vi "CAEN_HVBoard.ProcCases.vi"(0 "i ref in":refnum<vi>, 1 "selector":string, 2 "Data":T1, 3 "call cluster":T2={"Object"="", "Selector"="", "CallType"=enum."synchronous", "Async Object"="", "Async Selector"="", "Data Descriptor"="", "Data"=[], "Error #"=0, "Expire"=0}, 5 "error in (no error)":errorcluster) -> (14 "i ref out":refnum<vi>, 17 "answer cluster":T2={"Object"="", "Selector"="", "CallType"=enum."synchronous", "Async Object"="", "Async Selector"="", "Data Descriptor"="", "Data"=[], "Error #"=0, "Expire"=0}, 19 "error out":errorcluster)   [LabVIEW 2014, in "CAEN_HVBoard.lvlib"]
doc: "This method is called by a process from within the default case in the event loop. The methods of a class that are linked to events will be called from THIS method. Add your code here."
uses:
  CAEN_HVBoard.lvlib
  CSCore/CSSystem/CoreDefs/CoreDefs.call_type.ctl
  CSCore/BaseProcess/BaseProcess.descriptor string definition.ctl
  CSCore/CSSystem/CoreDefs/CoreDefs.rawDataType.ctl
  CSCore/CSApplicationBaseClasses/DeviceBase/DeviceBase.deviceState.ctl
  CSCore/CSSystem/CoreLib/CoreLib.string 2 byte array.vi
  CSCore/CSSystem/CoreLib/CoreLib.byte array 2 string.vi
  CSCore/CSSystem/CoreLib/CoreLib.lvlib
  CSCore/BaseProcess/BaseProcess.lvlib
  CSCore/CSApplicationBaseClasses/DeviceBase/DeviceBase.lvlib
  CSCore/CAEObj/CAEObj.lvlib
  CAEN_HVSystem/CAEN_HVSystem.lvlib
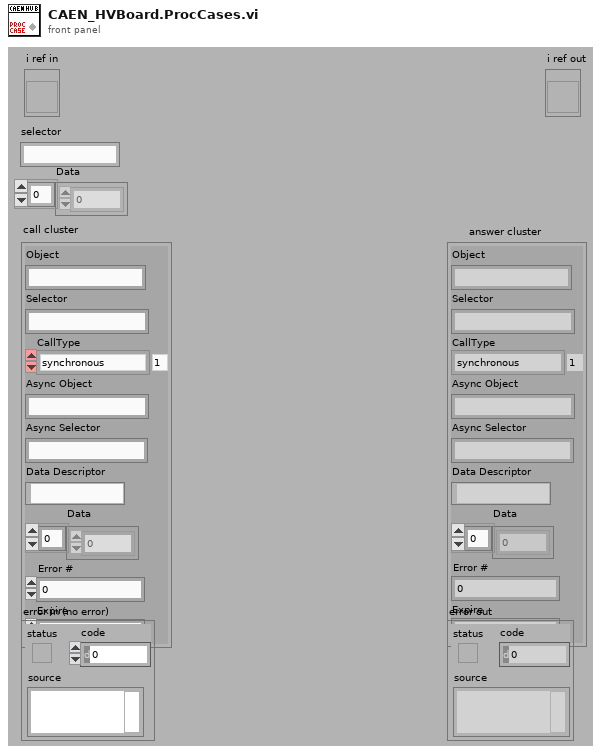
[diagram p1: front panel]
types:
  T1 = typedef "CoreDefs.rawDataType.ctl" = i8[]
  T2 = typedef "CoreDefs.call_type.ctl" = cluster{"Object":string, "Selector":string, "CallType":enum16{"simple", "synchronous", "asynchronous"}, "Async Object":string, "Async Selector":string, "Data Descriptor":T3, "Data":T1, "Error #":i32, "Expire":u32}
  T3 = typedef "BaseProcess.lvlib/BaseProcess.descriptor string definition.ctl" = string
  T4 = typedef "CAEN_HVBoard.lvlib/CAEN_HVBoard.i attribute.ctl" = cluster{"System Name":string, "Board ID":i32, "Prefix":string, "HVMaxMultiplier":dbl, "Temp#Multiplier":dbl, "Model Name":cluster{"Model Name":string, "DIM Status":cluster{"no link":bool, "quality":i32, "Time Stamp":timestamp}}, "Description":cluster{"Description":string, "DIM Status":cluster{"no link":bool, "quality":i32, "Time Stamp":timestamp}}, "SerNum":cluster{"SerNum":i16, "DIM Status":cluster{"no link":bool, "quality":i32, "Time Stamp":timestamp}}, "NrOfCh":cluster{"NrOfCh":i16, "DIM Status":cluster{"no link":bool, "quality":i32, "Time Stamp":timestamp}}, "BdStatus":cluster{"BdStatus":i16, "DIM Status":cluster{"no link":bool, "quality":i32, "Time Stamp":timestamp}}, "HVMax":cluster{"HVMax":dbl, "DIM Status":cluster{"no link":bool, "quality":i32, "Time Stamp":timestamp}}, "HVMax#EU":cluster{"HVMax#EU":string, "DIM Status":cluster{"no link":bool, "quality":i32, "Time Stamp":timestamp}}, "HVMax#HighEU":cluster{"HVMax#HighEU":dbl, "DIM Status":cluster{"no link":bool, "quality":i32, "Time Stamp":timestamp}}, "HVMax#LowEU":cluster{"HVMax#LowEU":dbl, "DIM Status":cluster{"no link":bool, "quality":i32, "Time Stamp":timestamp}}, "Temp#EU":cluster{"Temp#EU":string, "DIM Status":cluster{"no link":bool, "quality":i32, "Time Stamp":timestamp}}, "Temp":cluster{"Temp":dbl, "DIM Status":cluster{"no link":bool, "quality":i32, "Time Stamp":timestamp}}, "Temp#HighEU":cluster{"Temp#HighEU":dbl, "DIM Status":cluster{"no link":bool, "quality":i32, "Time Stamp":timestamp}}, "Temp#LowEU":cluster{"Temp#LowEU":dbl, "DIM Status":cluster{"no link":bool, "quality":i32, "Time Stamp":timestamp}}}
  T5 = typedef "DeviceBase.lvlib/DeviceBase.i attribute.ctl" = cluster{"deviceState":i32, "deviceStateID":i32, "deviceID":string, "deviceIDID":i32, "advancedGUIClass":string, "advancedGUIClassID":i32}
  T6 = typedef "DeviceBase.lvlib/DeviceBase.deviceState.ctl" = i16
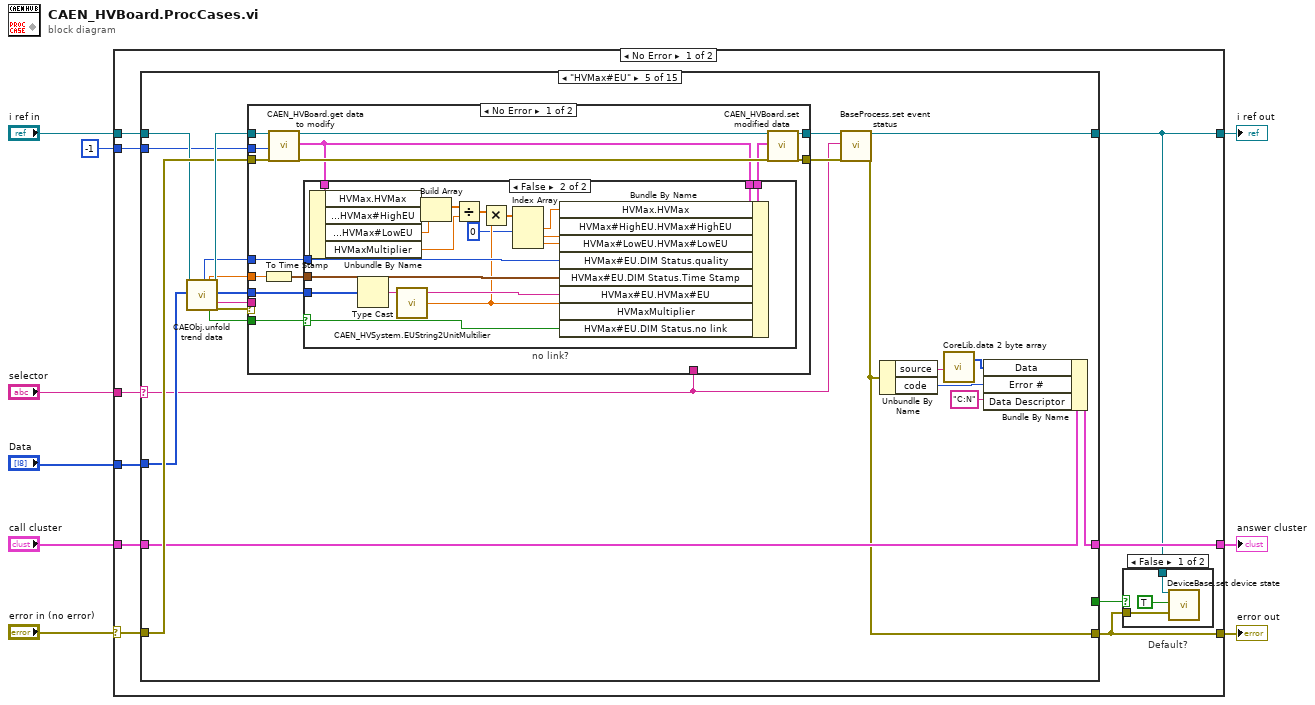
[diagram p0: block diagram]
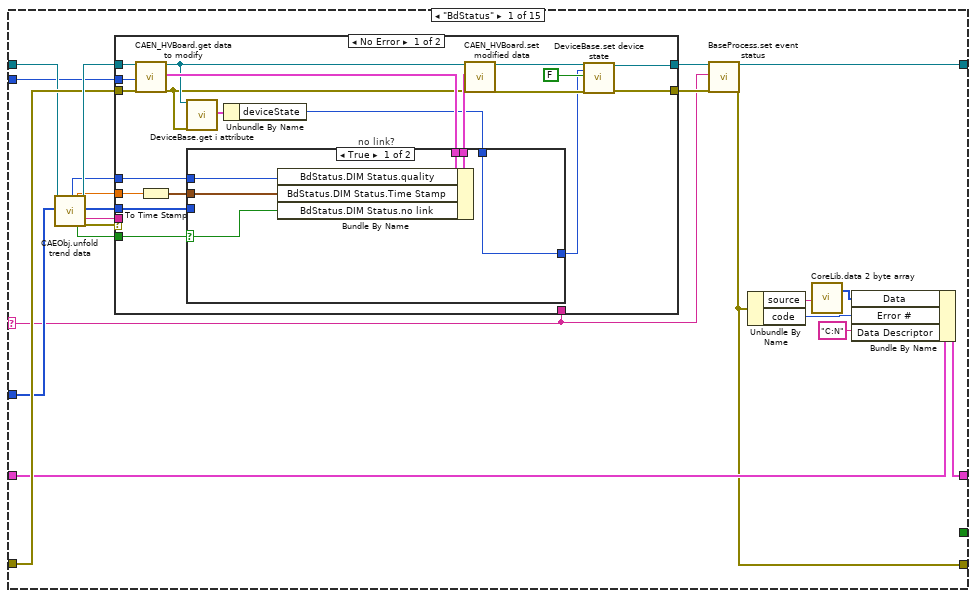
[diagram p3: hidden frame]
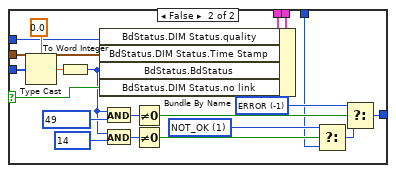
[diagram p4: hidden frame]
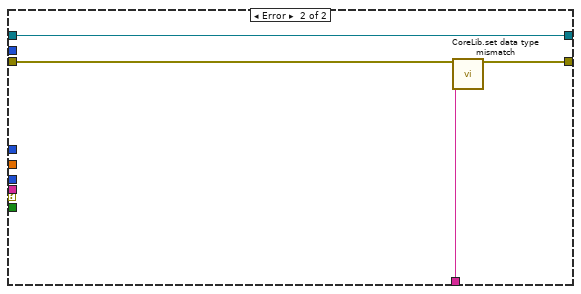
[diagram p5: hidden frame]
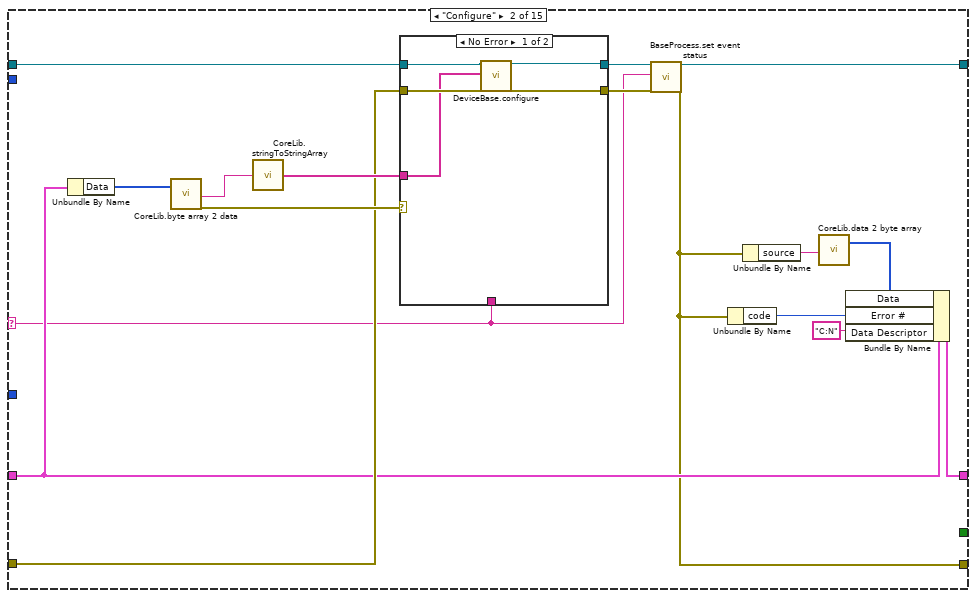
[diagram p6: hidden frame]
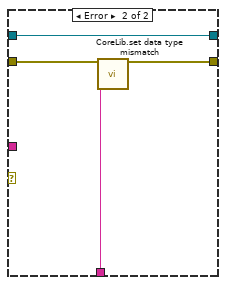
[diagram p7: hidden frame]
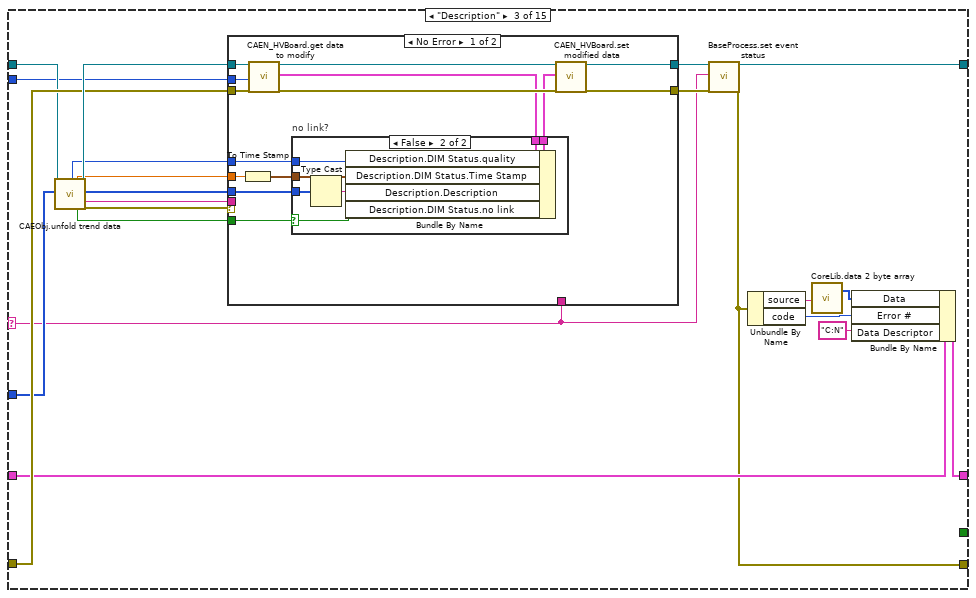
[diagram p8: hidden frame]
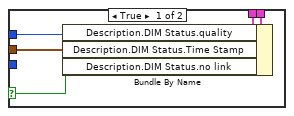
[diagram p9: hidden frame]
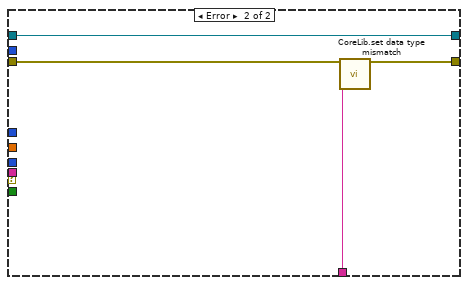
[diagram p10: hidden frame]
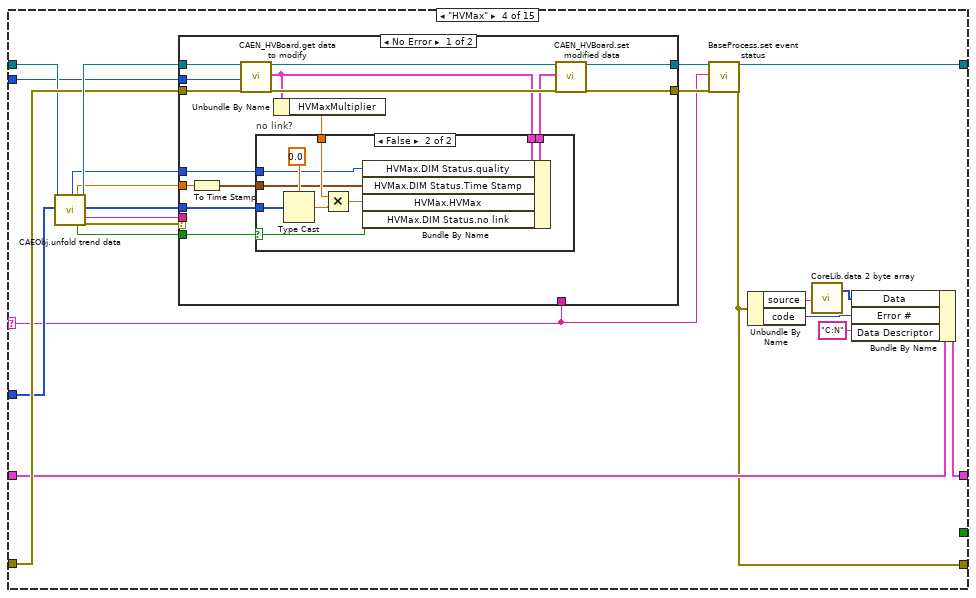
[diagram p11: hidden frame]
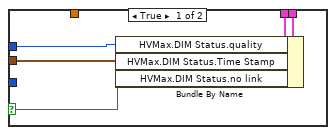
[diagram p12: hidden frame]
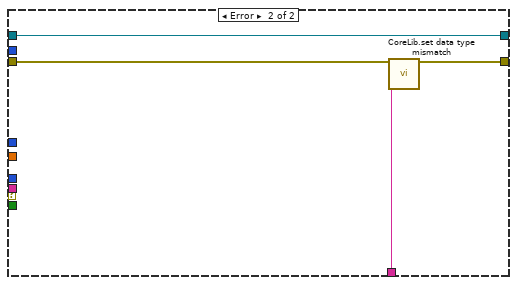
[diagram p13: hidden frame]
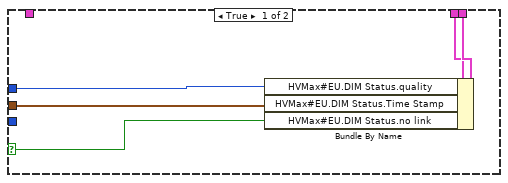
[diagram p14: hidden frame]
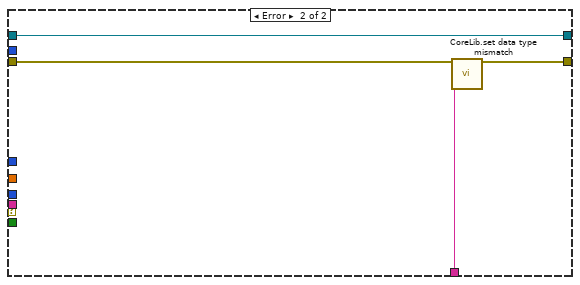
[diagram p15: hidden frame]
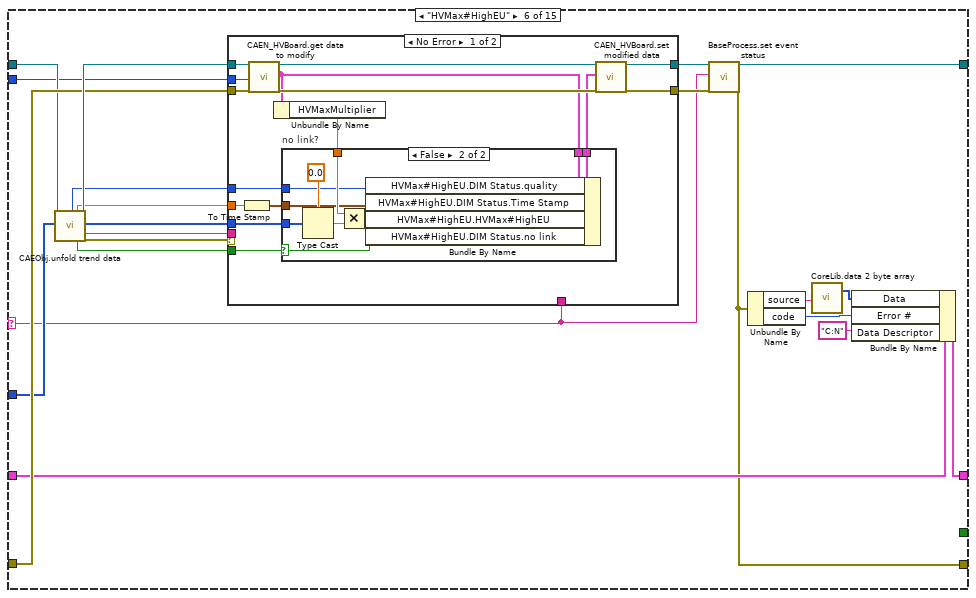
[diagram p16: hidden frame]
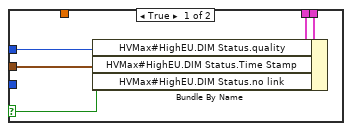
[diagram p17: hidden frame]
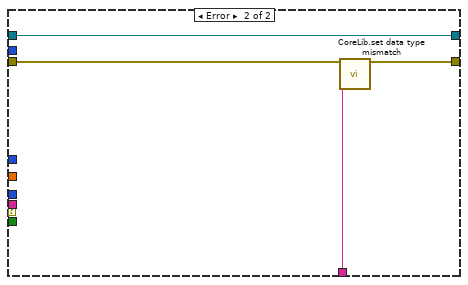
[diagram p18: hidden frame]
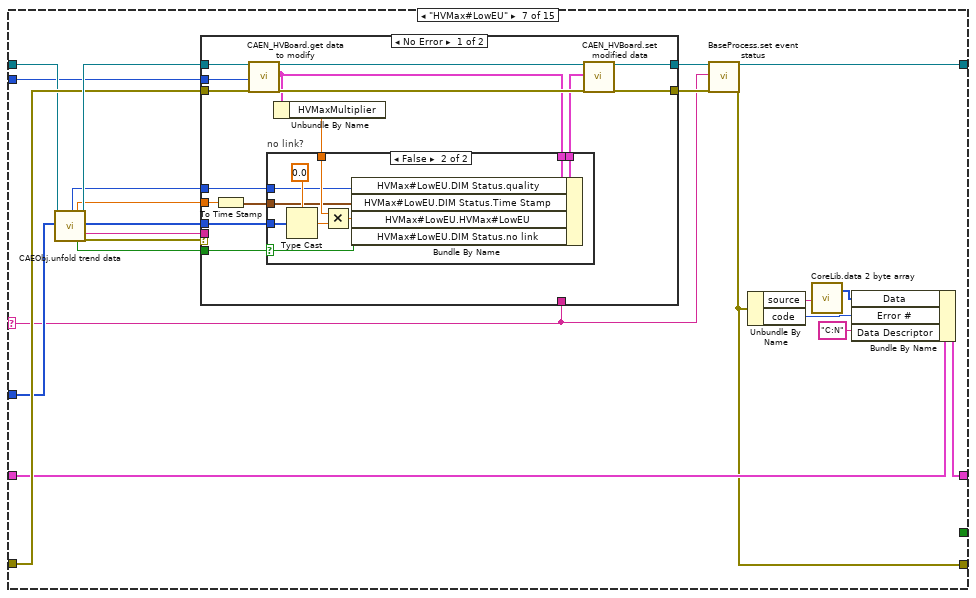
[diagram p19: hidden frame]
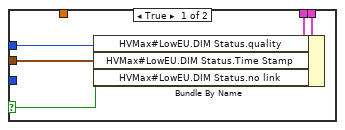
[diagram p20: hidden frame]
diagram:
  n1 = case shown="No Error" "error in (no error)" {
    selector: "error in (no error)" -> [w14 w848]
    tunnel: "selector" -> [w19 _]
    tunnel: [w18 w849] -> w8
    tunnel: "Data" -> [w17 _]
    tunnel: "call cluster" -> [w16 w849]
    tunnel: "i ref in" -> [w15 w850]
    tunnel: [w10 w850] -> w4
    tunnel: [w12 w848] -> w3
    tunnel: -1 ("ms timeout (10000)") -> [w11 _]
    frame No Error {
      n2 = case shown="\"HVMax#EU\"" w19 {
        selector: w19 -> [w32 w99 w129 w181 w237 w303 w359 w415 w487 w541 w615 w671 w737 w793 w842]
        tunnel: w17 -> [w33 _ w130 w182 w238 w304 w360 w416 w488 w542 w616 w672 w738 w794 _]
        tunnel: w15 -> [w31 w98 w128 w180 w236 w302 w358 w414 w486 w540 w614 w670 w736 w792 w841]
        tunnel: [w27 w97 w124 w176 w232 w298 w354 w410 w482 w536 w610 w666 w732 w788 w847] -> w10
        tunnel: w16 -> [w34 w100 w131 w183 w239 w305 w361 w417 w489 w543 w617 w673 w739 w795 w843]
        tunnel: [w28 w96 w125 w177 w233 w299 w355 w411 w483 w537 w611 w667 w733 w789 w844] -> w18
        tunnel: w14 -> [w35 w101 w132 w184 w240 w306 w362 w418 w490 w544 w618 w674 w740 w796 w846]
        tunnel: [w29 w95 w126 w178 w234 w300 w356 w412 w484 w538 w612 w668 w734 w790 w845] -> w12
        tunnel: [_ _ _ _ _ _ _ _ _ _ _ _ _ _ TRUE] -> w13
        tunnel: w11 -> [w30 _ w127 w179 w235 w301 w357 w413 w485 w539 w613 w669 w735 w791 _]
        frame "BdStatus" {
          n3 = call "CAEObj.unfold trend data.vi"("i ref in"=w31, "raw trend data"=w33) -> ("quality"=w26:i32, "timeStamp"=w25:dbl, "no link"=w23:bool, "i ref out"=w39:refnum<vi>, "data"=w38:i8[], "typeDescriptor"=w36:string, "error out"=w24:errorcluster)  [unwired: 9 in, 2 out]
          n4 = case shown="No Error" w24 {
            tunnel: [w48 w94] -> w42
            tunnel: w39 -> [w64 w94]
            tunnel: w35 -> [w63 w93]
            tunnel: [w47 w92] -> w41
            tunnel: w32 -> [_ w91]
            tunnel: w30 -> [w62 _]
            tunnel: w38 -> [w60 _]
            tunnel: w36 -> [_ _]
            tunnel: w26 -> [w58 _]
            tunnel: w25 -> [w56 _]
            tunnel: w23 -> [w55 _]
            frame No Error {
              n5 = call "CAEN_HVBoard.get data to modify.vi"("i ref in"=w64, "ms timeout (10000)"=w62, "error in (no error)"=w63) -> ("i ref out"=w53:refnum<vi>, "i attribute"=w59:T4, "error out"=w52:errorcluster)  [unwired: 13 in, 1 out]
              n6 = To Time Stamp(1:w56) -> (0:w57:timestamp)
              n7 = call "DeviceBase.get i attribute.vi"("i ref in"=w53, "error in (no error)"=w52) -> ("i attribute"=w54:T5)  [unwired: 15 in, 2 out]
              n8 = Unbundle By Name(w54) -> ("deviceState"=w45:i32)
              n9 = case "no link?" shown="True" w55 {
                selector: w55 -> [w66 w83]
                tunnel: [w70 w90] -> w61
                tunnel: w60 -> [_ w89]
                tunnel: w59 -> [w69 w88]
                tunnel: w58 -> [w68 w85]
                tunnel: w57 -> [w67 w84]
                tunnel: [w65 w79] -> w46
                tunnel: w45 -> [w65 w71]
                frame True {
                  n10 = Bundle By Name(cluster=w69, "BdStatus.DIM Status.quality"=w68, "BdStatus.DIM Status.Time Stamp"=w67, "BdStatus.DIM Status.no link"=w66) -> (w70:T4)
                }
                frame False {
                  w73 = T6 1 items=["ERROR"=-1, "OK"=0, "NOT_OK"=1] ("deviceState")
                  w82 = T6 -1 items=["ERROR"=-1, "OK"=0, "NOT_OK"=1] ("deviceState")
                  n11 = Type Cast(type=0.0, x=w89) -> (*(type *) &x=w87:dbl)
                  n12 = To Word Integer(number=w87) -> (16bit integer=w76:i16)
                  n13 = Bundle By Name(cluster=w88, "BdStatus.DIM Status.quality"=w85, "BdStatus.DIM Status.Time Stamp"=w84, "BdStatus.BdStatus"=w76, "BdStatus.DIM Status.no link"=w83) -> (w90:T4)
                  n14 = And(x=w76, y=i16 49) -> (x .and. y?=w81:i16)
                  n15 = And(x=w76, y=i16 14) -> (x .and. y?=w78:i16)
                  n16 = Not Equal To 0?(x=w81) -> (x != 0?=w80:bool)
                  n17 = Not Equal To 0?(x=w78) -> (x != 0?=w74:bool)
                  n18 = Select(t=w73, s=w74, f=w71) -> (s? t:f=w72:i32)
                  n19 = Select(t=w82, s=w80, f=w72) -> (s? t:f=w79:i32)
                }
              }
              n20 = call "CAEN_HVBoard.set modified data.vi"("i ref in"=w53, "i attribute"=w61, "error in (no error)"=w52) -> ("i ref out"=w49:refnum<vi>, "error out"=w50:errorcluster)  [unwired: 15 in]
              n21 = call "DeviceBase.set device state.vi"("i ref in"=w49, "deviceState"=w46, "implicit"=FALSE, "error in (no error)"=w50) -> ("i ref out"=w48:refnum<vi>, "error out"=w47:errorcluster)  [unwired: 13 in, 1 out]
            }
            frame Error {
              n22 = call "CoreLib.set data type mismatch.vi"("error in (no error)"=w93, "error source"=w91) -> ("error out"=w92:errorcluster)  [unwired: 17 in]
            }
          }
          n23 = call "BaseProcess.set event status.vi"("i ref in"=w42, "EventStatus"=w32, "error in (no error)"=w41) -> ("i ref out"=w27:refnum<vi>, "error out"=w29:errorcluster)  [unwired: 14 in, 1 out]
          n24 = Unbundle By Name(w29) -> ("source"=w37:string, "code"=w44:i32)
          n25 = call-poly "CoreLib.data 2 byte array.vi"("string"=w37) -> ("byteArray out"=w43:T1)  [unwired: 18 in]
          n26 = Bundle By Name(cluster=w34, "Data"=w43, "Error #"=w44, "Data Descriptor"="C:N") -> (w28:T2)
        }
        frame "Configure" {
          n27 = Unbundle By Name(w100) -> ("Data"=w106:T1)
          n28 = call-poly "CoreLib.byte array 2 data.vi"("byteArray"=w106) -> ("string"=w103:string, "error out"=w104:errorcluster)  [unwired: 16 in, 1 out]
          n29 = call "CoreLib.stringToStringArray.vi"("String"=w103) -> ("Array"=w102:string[])
          n30 = case shown="No Error" w104 {
            tunnel: [w113 w119] -> w109
            tunnel: w98 -> [w114 w119]
            tunnel: w101 -> [w115 w118]
            tunnel: [w115 w117] -> w108
            tunnel: w99 -> [_ w116]
            tunnel: w102 -> [w112 _]
            frame No Error {
              n31 = call "DeviceBase.configure.vi"("i ref in"=w114, "configureData"=w112) -> ("i ref out"=w113:refnum<vi>)  [unwired: 15 in, 2 out]
            }
            frame Error {
              n32 = call "CoreLib.set data type mismatch.vi"("error in (no error)"=w118, "error source"=w116) -> ("error out"=w117:errorcluster)  [unwired: 17 in]
            }
          }
          n33 = call "BaseProcess.set event status.vi"("i ref in"=w109, "EventStatus"=w99, "error in (no error)"=w108) -> ("i ref out"=w97:refnum<vi>, "error out"=w95:errorcluster)  [unwired: 14 in, 1 out]
          n34 = Unbundle By Name(w95) -> ("code"=w111:i32)
          n35 = Unbundle By Name(w95) -> ("source"=w105:string)
          n36 = call-poly "CoreLib.data 2 byte array.vi"("string"=w105) -> ("byteArray out"=w110:T1)  [unwired: 18 in]
          n37 = Bundle By Name(cluster=w100, "Data"=w110, "Error #"=w111, "Data Descriptor"="C:N") -> (w96:T2)
        }
        frame "Description" {
          n38 = call "CAEObj.unfold trend data.vi"("i ref in"=w128, "raw trend data"=w130) -> ("quality"=w123:i32, "timeStamp"=w122:dbl, "no link"=w120:bool, "i ref out"=w136:refnum<vi>, "data"=w135:i8[], "typeDescriptor"=w133:string, "error out"=w121:errorcluster)  [unwired: 9 in, 2 out]
          n39 = case shown="No Error" w121 {
            tunnel: [w147 w171] -> w139
            tunnel: w136 -> [w155 w171]
            tunnel: w132 -> [w154 w170]
            tunnel: [w146 w169] -> w138
            tunnel: w129 -> [_ w168]
            tunnel: w127 -> [w153 _]
            tunnel: w135 -> [w149 _]
            tunnel: w133 -> [_ _]
            tunnel: w123 -> [w145 _]
            tunnel: w122 -> [w144 _]
            tunnel: w120 -> [w142 _]
            frame No Error {
              n40 = To Time Stamp(1:w144) -> (0:w143:timestamp)
              n41 = call "CAEN_HVBoard.get data to modify.vi"("i ref in"=w155, "ms timeout (10000)"=w153, "error in (no error)"=w154) -> ("i ref out"=w152:refnum<vi>, "i attribute"=w148:T4, "error out"=w151:errorcluster)  [unwired: 13 in, 1 out]
              n42 = case "no link?" shown="False" w142 {
                selector: w142 -> [w156 w161]
                tunnel: [w160 w167] -> w150
                tunnel: w149 -> [_ w166]
                tunnel: w148 -> [w159 w165]
                tunnel: w145 -> [w158 w163]
                tunnel: w143 -> [w157 w162]
                frame True {
                  n43 = Bundle By Name(cluster=w159, "Description.DIM Status.quality"=w158, "Description.DIM Status.Time Stamp"=w157, "Description.DIM Status.no link"=w156) -> (w160:T4)
                }
                frame False {
                  n44 = Type Cast(x=w166) -> (*(type *) &x=w164:string)  [unwired: 1 in]
                  n45 = Bundle By Name(cluster=w165, "Description.DIM Status.quality"=w163, "Description.DIM Status.Time Stamp"=w162, "Description.Description"=w164, "Description.DIM Status.no link"=w161) -> (w167:T4)
                }
              }
              n46 = call "CAEN_HVBoard.set modified data.vi"("i ref in"=w152, "i attribute"=w150, "error in (no error)"=w151) -> ("i ref out"=w147:refnum<vi>, "error out"=w146:errorcluster)  [unwired: 15 in]
            }
            frame Error {
              n47 = call "CoreLib.set data type mismatch.vi"("error in (no error)"=w170, "error source"=w168) -> ("error out"=w169:errorcluster)  [unwired: 17 in]
            }
          }
          n48 = call "BaseProcess.set event status.vi"("i ref in"=w139, "EventStatus"=w129, "error in (no error)"=w138) -> ("i ref out"=w124:refnum<vi>, "error out"=w126:errorcluster)  [unwired: 14 in, 1 out]
          n49 = Unbundle By Name(w126) -> ("source"=w134:string, "code"=w141:i32)
          n50 = call-poly "CoreLib.data 2 byte array.vi"("string"=w134) -> ("byteArray out"=w140:T1)  [unwired: 18 in]
          n51 = Bundle By Name(cluster=w131, "Data"=w140, "Error #"=w141, "Data Descriptor"="C:N") -> (w125:T2)
        }
        frame "HVMax" {
          n52 = call "CAEObj.unfold trend data.vi"("i ref in"=w180, "raw trend data"=w182) -> ("quality"=w175:i32, "timeStamp"=w174:dbl, "no link"=w172:bool, "i ref out"=w188:refnum<vi>, "data"=w187:i8[], "typeDescriptor"=w185:string, "error out"=w173:errorcluster)  [unwired: 9 in, 2 out]
          n53 = case shown="No Error" w173 {
            tunnel: [w201 w227] -> w191
            tunnel: w188 -> [w208 w227]
            tunnel: w184 -> [w207 w226]
            tunnel: [w200 w225] -> w190
            tunnel: w181 -> [_ w224]
            tunnel: w179 -> [w206 _]
            tunnel: w187 -> [w202 _]
            tunnel: w185 -> [_ _]
            tunnel: w175 -> [w197 _]
            tunnel: w174 -> [w195 _]
            tunnel: w172 -> [w194 _]
            frame No Error {
              n54 = To Time Stamp(1:w195) -> (0:w196:timestamp)
              n55 = call "CAEN_HVBoard.get data to modify.vi"("i ref in"=w208, "ms timeout (10000)"=w206, "error in (no error)"=w207) -> ("i ref out"=w205:refnum<vi>, "i attribute"=w199:T4, "error out"=w204:errorcluster)  [unwired: 13 in, 1 out]
              n56 = Unbundle By Name(w199) -> ("HVMaxMultiplier"=w198:dbl)
              n57 = case "no link?" shown="False" w194 {
                selector: w194 -> [w209 w214]
                tunnel: [w213 w223] -> w203
                tunnel: w202 -> [_ w222]
                tunnel: w199 -> [w212 w220]
                tunnel: w198 -> [_ w218]
                tunnel: w197 -> [w211 w216]
                tunnel: w196 -> [w210 w215]
                frame True {
                  n58 = Bundle By Name(cluster=w212, "HVMax.DIM Status.quality"=w211, "HVMax.DIM Status.Time Stamp"=w210, "HVMax.DIM Status.no link"=w209) -> (w213:T4)
                }
                frame False {
                  n59 = Type Cast(type=0.0, x=w222) -> (*(type *) &x=w219:dbl)
                  n60 = Multiply(x=w218, y=w219) -> (x*y=w217:dbl)
                  n61 = Bundle By Name(cluster=w220, "HVMax.DIM Status.quality"=w216, "HVMax.DIM Status.Time Stamp"=w215, "HVMax.HVMax"=w217, "HVMax.DIM Status.no link"=w214) -> (w223:T4)
                }
              }
              n62 = call "CAEN_HVBoard.set modified data.vi"("i ref in"=w205, "i attribute"=w203, "error in (no error)"=w204) -> ("i ref out"=w201:refnum<vi>, "error out"=w200:errorcluster)  [unwired: 15 in]
            }
            frame Error {
              n63 = call "CoreLib.set data type mismatch.vi"("error in (no error)"=w226, "error source"=w224) -> ("error out"=w225:errorcluster)  [unwired: 17 in]
            }
          }
          n64 = call "BaseProcess.set event status.vi"("i ref in"=w191, "EventStatus"=w181, "error in (no error)"=w190) -> ("i ref out"=w176:refnum<vi>, "error out"=w178:errorcluster)  [unwired: 14 in, 1 out]
          n65 = Unbundle By Name(w178) -> ("source"=w186:string, "code"=w193:i32)
          n66 = call-poly "CoreLib.data 2 byte array.vi"("string"=w186) -> ("byteArray out"=w192:T1)  [unwired: 18 in]
          n67 = Bundle By Name(cluster=w183, "Data"=w192, "Error #"=w193, "Data Descriptor"="C:N") -> (w177:T2)
        }
        frame "HVMax#EU" {
          n68 = call "CAEObj.unfold trend data.vi"("i ref in"=w236, "raw trend data"=w238) -> ("quality"=w230:i32, "timeStamp"=w229:dbl, "no link"=w228:bool, "i ref out"=w244:refnum<vi>, "data"=w243:i8[], "typeDescriptor"=w241:string, "error out"=w231:errorcluster)  [unwired: 9 in, 2 out]
          n69 = case shown="No Error" w231 {
            tunnel: [w256 w293] -> w247
            tunnel: w244 -> [w263 w293]
            tunnel: w240 -> [w262 w292]
            tunnel: [w255 w291] -> w246
            tunnel: w237 -> [_ w290]
            tunnel: w235 -> [w261 _]
            tunnel: w243 -> [w257 _]
            tunnel: w241 -> [_ _]
            tunnel: w230 -> [w254 _]
            tunnel: w229 -> [w252 _]
            tunnel: w228 -> [w251 _]
            frame No Error {
              n70 = To Time Stamp(1:w252) -> (0:w253:timestamp)
              n71 = call "CAEN_HVBoard.get data to modify.vi"("i ref in"=w263, "ms timeout (10000)"=w261, "error in (no error)"=w262) -> ("i ref out"=w260:refnum<vi>, "i attribute"=w250:T4, "error out"=w259:errorcluster)  [unwired: 13 in, 1 out]
              n72 = case "no link?" shown="False" w251 {
                selector: w251 -> [w264 w282]
                tunnel: [w268 w289] -> w258
                tunnel: w257 -> [_ w288]
                tunnel: w250 -> [w267 w287]
                tunnel: w254 -> [w266 w284]
                tunnel: w253 -> [w265 w283]
                tunnel: w250 -> [_ w281]
                frame True {
                  n73 = Bundle By Name(cluster=w267, "HVMax#EU.DIM Status.quality"=w266, "HVMax#EU.DIM Status.Time Stamp"=w265, "HVMax#EU.DIM Status.no link"=w264) -> (w268:T4)
                }
                frame False {
                  n74 = Unbundle By Name(w281) -> ("HVMax.HVMax"=w278:dbl, "HVMax#HighEU.HVMax#HighEU"=w277:dbl, "HVMax#LowEU.HVMax#LowEU"=w276:dbl, "HVMaxMultiplier"=w274:dbl)
                  n75 = Type Cast(x=w288) -> (*(type *) &x=w286:string)  [unwired: 1 in]
                  n76 = call "CAEN_HVSystem.EUString2UnitMultilier.vi"("EU String"=w286) -> ("Multiplier"=w279:dbl, "Unit"=w285:string)  [unwired: 2 in, 1 out]
                  n77 = Build Array(w278, w277, w276) -> (w275:dbl[])
                  n78 = Divide(x=w275, y=w274) -> (x/y=w280:dbl[])
                  n79 = Multiply(x=w280, y=w279) -> (x*y=w273:dbl[])
                  n80 = Index Array(array=w273, index #1=0 ("index")) -> (element #1=w271:dbl, element #2=w270:dbl, element #3=w269:dbl)  [unwired: 2 in]
                  n81 = Bundle By Name(cluster=w287, "HVMax.HVMax"=w271, "HVMax#HighEU.HVMax#HighEU"=w270, "HVMax#LowEU.HVMax#LowEU"=w269, "HVMax#EU.DIM Status.quality"=w284, "HVMax#EU.DIM Status.Time Stamp"=w283, "HVMax#EU.HVMax#EU"=w285, "HVMaxMultiplier"=w279, "HVMax#EU.DIM Status.no link"=w282) -> (w289:T4)
                }
              }
              n82 = call "CAEN_HVBoard.set modified data.vi"("i ref in"=w260, "i attribute"=w258, "error in (no error)"=w259) -> ("i ref out"=w256:refnum<vi>, "error out"=w255:errorcluster)  [unwired: 15 in]
            }
            frame Error {
              n83 = call "CoreLib.set data type mismatch.vi"("error in (no error)"=w292, "error source"=w290) -> ("error out"=w291:errorcluster)  [unwired: 17 in]
            }
          }
          n84 = call "BaseProcess.set event status.vi"("i ref in"=w247, "EventStatus"=w237, "error in (no error)"=w246) -> ("i ref out"=w232:refnum<vi>, "error out"=w234:errorcluster)  [unwired: 14 in, 1 out]
          n85 = Unbundle By Name(w234) -> ("source"=w242:string, "code"=w249:i32)
          n86 = call-poly "CoreLib.data 2 byte array.vi"("string"=w242) -> ("byteArray out"=w248:T1)  [unwired: 18 in]
          n87 = Bundle By Name(cluster=w239, "Data"=w248, "Error #"=w249, "Data Descriptor"="C:N") -> (w233:T2)
        }
        frame "HVMax#HighEU" {
          n88 = call "CAEObj.unfold trend data.vi"("i ref in"=w302, "raw trend data"=w304) -> ("quality"=w296:i32, "timeStamp"=w295:dbl, "no link"=w294:bool, "i ref out"=w310:refnum<vi>, "data"=w309:i8[], "typeDescriptor"=w307:string, "error out"=w297:errorcluster)  [unwired: 9 in, 2 out]
          n89 = case shown="No Error" w297 {
            tunnel: [w323 w349] -> w313
            tunnel: w310 -> [w330 w349]
            tunnel: w306 -> [w329 w348]
            tunnel: [w322 w347] -> w312
            tunnel: w303 -> [_ w346]
            tunnel: w301 -> [w328 _]
            tunnel: w309 -> [w324 _]
            tunnel: w307 -> [_ _]
            tunnel: w296 -> [w319 _]
            tunnel: w295 -> [w318 _]
            tunnel: w294 -> [w316 _]
            frame No Error {
              n90 = To Time Stamp(1:w318) -> (0:w317:timestamp)
              n91 = call "CAEN_HVBoard.get data to modify.vi"("i ref in"=w330, "ms timeout (10000)"=w328, "error in (no error)"=w329) -> ("i ref out"=w327:refnum<vi>, "i attribute"=w321:T4, "error out"=w326:errorcluster)  [unwired: 13 in, 1 out]
              n92 = Unbundle By Name(w321) -> ("HVMaxMultiplier"=w320:dbl)
              n93 = case "no link?" shown="False" w316 {
                selector: w316 -> [w331 w336]
                tunnel: [w335 w345] -> w325
                tunnel: w324 -> [_ w344]
                tunnel: w321 -> [w334 w342]
                tunnel: w320 -> [_ w340]
                tunnel: w319 -> [w333 w338]
                tunnel: w317 -> [w332 w337]
                frame True {
                  n94 = Bundle By Name(cluster=w334, "HVMax#HighEU.DIM Status.quality"=w333, "HVMax#HighEU.DIM Status.Time Stamp"=w332, "HVMax#HighEU.DIM Status.no link"=w331) -> (w335:T4)
                }
                frame False {
                  n95 = Type Cast(type=0.0, x=w344) -> (*(type *) &x=w341:dbl)
                  n96 = Multiply(x=w340, y=w341) -> (x*y=w339:dbl)
                  n97 = Bundle By Name(cluster=w342, "HVMax#HighEU.DIM Status.quality"=w338, "HVMax#HighEU.DIM Status.Time Stamp"=w337, "HVMax#HighEU.HVMax#HighEU"=w339, "HVMax#HighEU.DIM Status.no link"=w336) -> (w345:T4)
                }
              }
              n98 = call "CAEN_HVBoard.set modified data.vi"("i ref in"=w327, "i attribute"=w325, "error in (no error)"=w326) -> ("i ref out"=w323:refnum<vi>, "error out"=w322:errorcluster)  [unwired: 15 in]
            }
            frame Error {
              n99 = call "CoreLib.set data type mismatch.vi"("error in (no error)"=w348, "error source"=w346) -> ("error out"=w347:errorcluster)  [unwired: 17 in]
            }
          }
          n100 = call "BaseProcess.set event status.vi"("i ref in"=w313, "EventStatus"=w303, "error in (no error)"=w312) -> ("i ref out"=w298:refnum<vi>, "error out"=w300:errorcluster)  [unwired: 14 in, 1 out]
          n101 = Unbundle By Name(w300) -> ("source"=w308:string, "code"=w315:i32)
          n102 = call-poly "CoreLib.data 2 byte array.vi"("string"=w308) -> ("byteArray out"=w314:T1)  [unwired: 18 in]
          n103 = Bundle By Name(cluster=w305, "Data"=w314, "Error #"=w315, "Data Descriptor"="C:N") -> (w299:T2)
        }
        frame "HVMax#LowEU" {
          n104 = call "CAEObj.unfold trend data.vi"("i ref in"=w358, "raw trend data"=w360) -> ("quality"=w352:i32, "timeStamp"=w351:dbl, "no link"=w350:bool, "i ref out"=w366:refnum<vi>, "data"=w365:i8[], "typeDescriptor"=w363:string, "error out"=w353:errorcluster)  [unwired: 9 in, 2 out]
          n105 = case shown="No Error" w353 {
            tunnel: [w379 w405] -> w369
            tunnel: w366 -> [w386 w405]
            tunnel: w362 -> [w385 w404]
            tunnel: [w378 w403] -> w368
            tunnel: w359 -> [_ w402]
            tunnel: w357 -> [w384 _]
            tunnel: w365 -> [w380 _]
            tunnel: w363 -> [_ _]
            tunnel: w352 -> [w375 _]
            tunnel: w351 -> [w373 _]
            tunnel: w350 -> [w372 _]
            frame No Error {
              n106 = To Time Stamp(1:w373) -> (0:w374:timestamp)
              n107 = call "CAEN_HVBoard.get data to modify.vi"("i ref in"=w386, "ms timeout (10000)"=w384, "error in (no error)"=w385) -> ("i ref out"=w383:refnum<vi>, "i attribute"=w377:T4, "error out"=w382:errorcluster)  [unwired: 13 in, 1 out]
              n108 = Unbundle By Name(w377) -> ("HVMaxMultiplier"=w376:dbl)
              n109 = case "no link?" shown="False" w372 {
                selector: w372 -> [w387 w392]
                tunnel: [w391 w401] -> w381
                tunnel: w380 -> [_ w400]
                tunnel: w377 -> [w390 w398]
                tunnel: w376 -> [_ w396]
                tunnel: w375 -> [w389 w394]
                tunnel: w374 -> [w388 w393]
                frame True {
                  n110 = Bundle By Name(cluster=w390, "HVMax#LowEU.DIM Status.quality"=w389, "HVMax#LowEU.DIM Status.Time Stamp"=w388, "HVMax#LowEU.DIM Status.no link"=w387) -> (w391:T4)
                }
                frame False {
                  n111 = Type Cast(type=0.0, x=w400) -> (*(type *) &x=w397:dbl)
                  n112 = Multiply(x=w396, y=w397) -> (x*y=w395:dbl)
                  n113 = Bundle By Name(cluster=w398, "HVMax#LowEU.DIM Status.quality"=w394, "HVMax#LowEU.DIM Status.Time Stamp"=w393, "HVMax#LowEU.HVMax#LowEU"=w395, "HVMax#LowEU.DIM Status.no link"=w392) -> (w401:T4)
                }
              }
              n114 = call "CAEN_HVBoard.set modified data.vi"("i ref in"=w383, "i attribute"=w381, "error in (no error)"=w382) -> ("i ref out"=w379:refnum<vi>, "error out"=w378:errorcluster)  [unwired: 15 in]
            }
            frame Error {
              n115 = call "CoreLib.set data type mismatch.vi"("error in (no error)"=w404, "error source"=w402) -> ("error out"=w403:errorcluster)  [unwired: 17 in]
            }
          }
          n116 = call "BaseProcess.set event status.vi"("i ref in"=w369, "EventStatus"=w359, "error in (no error)"=w368) -> ("i ref out"=w354:refnum<vi>, "error out"=w356:errorcluster)  [unwired: 14 in, 1 out]
          n117 = Unbundle By Name(w356) -> ("source"=w364:string, "code"=w371:i32)
          n118 = call-poly "CoreLib.data 2 byte array.vi"("string"=w364) -> ("byteArray out"=w370:T1)  [unwired: 18 in]
          n119 = Bundle By Name(cluster=w361, "Data"=w370, "Error #"=w371, "Data Descriptor"="C:N") -> (w355:T2)
        }
        frame "Model" {
          n120 = call "CAEObj.unfold trend data.vi"("i ref in"=w414, "raw trend data"=w416) -> ("quality"=w408:i32, "timeStamp"=w407:dbl, "no link"=w406:bool, "i ref out"=w422:refnum<vi>, "data"=w421:i8[], "typeDescriptor"=w419:string, "error out"=w409:errorcluster)  [unwired: 9 in, 2 out]
          n121 = case shown="No Error" w409 {
            tunnel: [w440 w477] -> w425
            tunnel: w422 -> [w447 w477]
            tunnel: w418 -> [w446 w476]
            tunnel: [w439 w475] -> w424
            tunnel: w415 -> [_ w474]
            tunnel: w413 -> [w445 _]
            tunnel: w421 -> [w441 _]
            tunnel: w419 -> [_ _]
            tunnel: w408 -> [w432 _]
            tunnel: w407 -> [w431 _]
            tunnel: w406 -> [w429 _]
            frame No Error {
              n122 = To Time Stamp(1:w431) -> (0:w430:timestamp)
              n123 = call "CAEN_HVBoard.get data to modify.vi"("i ref in"=w447, "ms timeout (10000)"=w445, "error in (no error)"=w446) -> ("i ref out"=w444:refnum<vi>, "i attribute"=w436:T4, "error out"=w443:errorcluster)  [unwired: 13 in, 1 out]
              n124 = Unbundle By Name(w436) -> ("Prefix"=w434:string, "SerNum.SerNum"=w433:i16)
              n125 = case "no link?" shown="False" w429 {
                selector: w429 -> [w448 w453]
                tunnel: [w452 w459] -> w442
                tunnel: w441 -> [_ w458]
                tunnel: w436 -> [w451 w457]
                tunnel: [_ w456] -> w435
                tunnel: w432 -> [w450 w455]
                tunnel: w430 -> [w449 w454]
                tunnel: [w448 w453] -> w428
                frame True {
                  n126 = Bundle By Name(cluster=w451, "Model Name.DIM Status.quality"=w450, "Model Name.DIM Status.Time Stamp"=w449, "Model Name.DIM Status.no link"=w448) -> (w452:T4)
                }
                frame False {
                  n127 = Type Cast(x=w458) -> (*(type *) &x=w456:string)  [unwired: 1 in]
                  n128 = Bundle By Name(cluster=w457, "Model Name.DIM Status.quality"=w455, "Model Name.DIM Status.Time Stamp"=w454, "Model Name.Model Name"=w456, "Model Name.DIM Status.no link"=w453) -> (w459:T4)
                }
              }
              n129 = call "CAEN_HVBoard.set modified data.vi"("i ref in"=w444, "i attribute"=w442, "error in (no error)"=w443) -> ("i ref out"=w437:refnum<vi>, "error out"=w438:errorcluster)  [unwired: 15 in]
              n130 = case "no link?" shown="False" w428 {
                tunnel: [w468 w473] -> w440
                tunnel: [w467 w472] -> w439
                tunnel: w438 -> [w466 w472]
                tunnel: w437 -> [w465 w473]
                tunnel: w435 -> [w464 _]
                tunnel: w434 -> [w463 _]
                tunnel: w433 -> [w461 _]
                frame False {
                  n131 = Number To Decimal String(number=w461) -> (decimal integer string=w460:string)  [unwired: 1 in]
                  n132 = Concatenate Strings("CAEN HV Board: " ("string"), w463, "; Model: " ("string"), w464, "; Serial number: " ("string"), w460) -> (w471:string)
                  n133 = call "DeviceBase.set device ID.vi"("i ref in"=w465, "deviceID"=w471, "error in (no error)"=w466) -> ("i ref out"=w468:refnum<vi>, "error out"=w467:errorcluster)  [unwired: 14 in, 1 out]
                }
                frame True {
                }
              }
            }
            frame Error {
              n134 = call "CoreLib.set data type mismatch.vi"("error in (no error)"=w476, "error source"=w474) -> ("error out"=w475:errorcluster)  [unwired: 17 in]
            }
          }
          n135 = call "BaseProcess.set event status.vi"("i ref in"=w425, "EventStatus"=w415, "error in (no error)"=w424) -> ("i ref out"=w410:refnum<vi>, "error out"=w412:errorcluster)  [unwired: 14 in, 1 out]
          n136 = Unbundle By Name(w412) -> ("source"=w420:string, "code"=w427:i32)
          n137 = call-poly "CoreLib.data 2 byte array.vi"("string"=w420) -> ("byteArray out"=w426:T1)  [unwired: 18 in]
          n138 = Bundle By Name(cluster=w417, "Data"=w426, "Error #"=w427, "Data Descriptor"="C:N") -> (w411:T2)
        }
        frame "NrOfCh" {
          n139 = call "CAEObj.unfold trend data.vi"("i ref in"=w486, "raw trend data"=w488) -> ("quality"=w480:i32, "timeStamp"=w479:dbl, "no link"=w478:bool, "i ref out"=w494:refnum<vi>, "data"=w493:i8[], "typeDescriptor"=w491:string, "error out"=w481:errorcluster)  [unwired: 9 in, 2 out]
          n140 = case shown="No Error" w481 {
            tunnel: [w505 w531] -> w497
            tunnel: w494 -> [w513 w531]
            tunnel: w490 -> [w512 w530]
            tunnel: [w504 w529] -> w496
            tunnel: w487 -> [_ w528]
            tunnel: w485 -> [w511 _]
            tunnel: w493 -> [w507 _]
            tunnel: w491 -> [_ _]
            tunnel: w480 -> [w503 _]
            tunnel: w479 -> [w502 _]
            tunnel: w478 -> [w500 _]
            frame No Error {
              n141 = To Time Stamp(1:w502) -> (0:w501:timestamp)
              n142 = call "CAEN_HVBoard.get data to modify.vi"("i ref in"=w513, "ms timeout (10000)"=w511, "error in (no error)"=w512) -> ("i ref out"=w510:refnum<vi>, "i attribute"=w506:T4, "error out"=w509:errorcluster)  [unwired: 13 in, 1 out]
              n143 = case "no link?" shown="False" w500 {
                selector: w500 -> [w514 w519]
                tunnel: [w518 w527] -> w508
                tunnel: w507 -> [_ w526]
                tunnel: w506 -> [w517 w525]
                tunnel: w503 -> [w516 w521]
                tunnel: w501 -> [w515 w520]
                frame True {
                  n144 = Bundle By Name(cluster=w517, "NrOfCh.DIM Status.quality"=w516, "NrOfCh.DIM Status.Time Stamp"=w515, "NrOfCh.DIM Status.no link"=w514) -> (w518:T4)
                }
                frame False {
                  n145 = Type Cast(type=0.0, x=w526) -> (*(type *) &x=w524:dbl)
                  n146 = To Word Integer(number=w524) -> (16bit integer=w522:i16)
                  n147 = Bundle By Name(cluster=w525, "NrOfCh.DIM Status.quality"=w521, "NrOfCh.DIM Status.Time Stamp"=w520, "NrOfCh.NrOfCh"=w522, "NrOfCh.DIM Status.no link"=w519) -> (w527:T4)
                }
              }
              n148 = call "CAEN_HVBoard.set modified data.vi"("i ref in"=w510, "i attribute"=w508, "error in (no error)"=w509) -> ("i ref out"=w505:refnum<vi>, "error out"=w504:errorcluster)  [unwired: 15 in]
            }
            frame Error {
              n149 = call "CoreLib.set data type mismatch.vi"("error in (no error)"=w530, "error source"=w528) -> ("error out"=w529:errorcluster)  [unwired: 17 in]
            }
          }
          n150 = call "BaseProcess.set event status.vi"("i ref in"=w497, "EventStatus"=w487, "error in (no error)"=w496) -> ("i ref out"=w482:refnum<vi>, "error out"=w484:errorcluster)  [unwired: 14 in, 1 out]
          n151 = Unbundle By Name(w484) -> ("source"=w492:string, "code"=w499:i32)
          n152 = call-poly "CoreLib.data 2 byte array.vi"("string"=w492) -> ("byteArray out"=w498:T1)  [unwired: 18 in]
          n153 = Bundle By Name(cluster=w489, "Data"=w498, "Error #"=w499, "Data Descriptor"="C:N") -> (w483:T2)
        }
        frame "SerNum" {
          n154 = call "CAEObj.unfold trend data.vi"("i ref in"=w540, "raw trend data"=w542) -> ("quality"=w533:i32, "timeStamp"=w532:dbl, "no link"=w534:bool, "i ref out"=w548:refnum<vi>, "data"=w547:i8[], "typeDescriptor"=w545:string, "error out"=w535:errorcluster)  [unwired: 9 in, 2 out]
          n155 = case shown="No Error" w535 {
            tunnel: [w566 w605] -> w551
            tunnel: w548 -> [w573 w605]
            tunnel: w544 -> [w572 w604]
            tunnel: [w565 w603] -> w550
            tunnel: w541 -> [_ w602]
            tunnel: w539 -> [w571 _]
            tunnel: w547 -> [w567 _]
            tunnel: w545 -> [_ _]
            tunnel: w534 -> [w554 _]
            tunnel: w533 -> [w558 _]
            tunnel: w532 -> [w556 _]
            frame No Error {
              n156 = To Time Stamp(1:w556) -> (0:w557:timestamp)
              n157 = call "CAEN_HVBoard.get data to modify.vi"("i ref in"=w573, "ms timeout (10000)"=w571, "error in (no error)"=w572) -> ("i ref out"=w570:refnum<vi>, "i attribute"=w562:T4, "error out"=w569:errorcluster)  [unwired: 13 in, 1 out]
              n158 = case "no link?" shown="False" w554 {
                selector: w554 -> [w574 w579]
                tunnel: [w578 w587] -> w568
                tunnel: w567 -> [_ w586]
                tunnel: w562 -> [w577 w583]
                tunnel: [_ w582] -> w559
                tunnel: w558 -> [w576 w581]
                tunnel: w557 -> [w575 w580]
                tunnel: [w574 w579] -> w555
                frame True {
                  n159 = Bundle By Name(cluster=w577, "SerNum.DIM Status.quality"=w576, "SerNum.DIM Status.Time Stamp"=w575, "SerNum.DIM Status.no link"=w574) -> (w578:T4)
                }
                frame False {
                  n160 = Type Cast(type=0.0, x=w586) -> (*(type *) &x=w585:dbl)
                  n161 = To Word Integer(number=w585) -> (16bit integer=w582:i16)
                  n162 = Bundle By Name(cluster=w583, "SerNum.DIM Status.quality"=w581, "SerNum.DIM Status.Time Stamp"=w580, "SerNum.SerNum"=w582, "SerNum.DIM Status.no link"=w579) -> (w587:T4)
                }
              }
              n163 = Unbundle By Name(w562) -> ("Prefix"=w561:string, "Model Name.Model Name"=w560:string)
              n164 = call "CAEN_HVBoard.set modified data.vi"("i ref in"=w570, "i attribute"=w568, "error in (no error)"=w569) -> ("i ref out"=w563:refnum<vi>, "error out"=w564:errorcluster)  [unwired: 15 in]
              n165 = case "no link?" shown="False" w555 {
                tunnel: [w596 w601] -> w566
                tunnel: [w595 w600] -> w565
                tunnel: w564 -> [w594 w600]
                tunnel: w563 -> [w593 w601]
                tunnel: w561 -> [w592 _]
                tunnel: w560 -> [w589 _]
                tunnel: w559 -> [w588 _]
                frame False {
                  n166 = Number To Decimal String(number=w588) -> (decimal integer string=w590:string)  [unwired: 1 in]
                  n167 = Concatenate Strings("CAEN HV Board: " ("string"), w592, "; Model: " ("string"), w589, "; Serial number: " ("string"), w590) -> (w599:string)
                  n168 = call "DeviceBase.set device ID.vi"("i ref in"=w593, "deviceID"=w599, "error in (no error)"=w594) -> ("i ref out"=w596:refnum<vi>, "error out"=w595:errorcluster)  [unwired: 14 in, 1 out]
                }
                frame True {
                }
              }
            }
            frame Error {
              n169 = call "CoreLib.set data type mismatch.vi"("error in (no error)"=w604, "error source"=w602) -> ("error out"=w603:errorcluster)  [unwired: 17 in]
            }
          }
          n170 = call "BaseProcess.set event status.vi"("i ref in"=w551, "EventStatus"=w541, "error in (no error)"=w550) -> ("i ref out"=w536:refnum<vi>, "error out"=w538:errorcluster)  [unwired: 14 in, 1 out]
          n171 = Unbundle By Name(w538) -> ("source"=w546:string, "code"=w553:i32)
          n172 = call-poly "CoreLib.data 2 byte array.vi"("string"=w546) -> ("byteArray out"=w552:T1)  [unwired: 18 in]
          n173 = Bundle By Name(cluster=w543, "Data"=w552, "Error #"=w553, "Data Descriptor"="C:N") -> (w537:T2)
        }
        frame "Temp" {
          n174 = call "CAEObj.unfold trend data.vi"("i ref in"=w614, "raw trend data"=w616) -> ("quality"=w608:i32, "timeStamp"=w607:dbl, "no link"=w606:bool, "i ref out"=w622:refnum<vi>, "data"=w621:i8[], "typeDescriptor"=w619:string, "error out"=w609:errorcluster)  [unwired: 9 in, 2 out]
          n175 = case shown="No Error" w609 {
            tunnel: [w635 w661] -> w625
            tunnel: w622 -> [w642 w661]
            tunnel: w618 -> [w641 w660]
            tunnel: [w634 w659] -> w624
            tunnel: w615 -> [_ w658]
            tunnel: w613 -> [w640 _]
            tunnel: w621 -> [w636 _]
            tunnel: w619 -> [_ _]
            tunnel: w608 -> [w631 _]
            tunnel: w607 -> [w629 _]
            tunnel: w606 -> [w628 _]
            frame No Error {
              n176 = To Time Stamp(1:w629) -> (0:w630:timestamp)
              n177 = call "CAEN_HVBoard.get data to modify.vi"("i ref in"=w642, "ms timeout (10000)"=w640, "error in (no error)"=w641) -> ("i ref out"=w639:refnum<vi>, "i attribute"=w633:T4, "error out"=w638:errorcluster)  [unwired: 13 in, 1 out]
              n178 = Unbundle By Name(w633) -> ("Temp#Multiplier"=w632:dbl)
              n179 = case "no link?" shown="False" w628 {
                selector: w628 -> [w643 w648]
                tunnel: [w647 w657] -> w637
                tunnel: w636 -> [_ w656]
                tunnel: w633 -> [w646 w654]
                tunnel: w632 -> [_ w652]
                tunnel: w631 -> [w645 w650]
                tunnel: w630 -> [w644 w649]
                frame True {
                  n180 = Bundle By Name(cluster=w646, "Temp.DIM Status.quality"=w645, "Temp.DIM Status.Time Stamp"=w644, "Temp.DIM Status.no link"=w643) -> (w647:T4)
                }
                frame False {
                  n181 = Type Cast(type=0.0, x=w656) -> (*(type *) &x=w653:dbl)
                  n182 = Multiply(x=w652, y=w653) -> (x*y=w651:dbl)
                  n183 = Bundle By Name(cluster=w654, "Temp.DIM Status.quality"=w650, "Temp.DIM Status.Time Stamp"=w649, "Temp.Temp"=w651, "Temp.DIM Status.no link"=w648) -> (w657:T4)
                }
              }
              n184 = call "CAEN_HVBoard.set modified data.vi"("i ref in"=w639, "i attribute"=w637, "error in (no error)"=w638) -> ("i ref out"=w635:refnum<vi>, "error out"=w634:errorcluster)  [unwired: 15 in]
            }
            frame Error {
              n185 = call "CoreLib.set data type mismatch.vi"("error in (no error)"=w660, "error source"=w658) -> ("error out"=w659:errorcluster)  [unwired: 17 in]
            }
          }
          n186 = call "BaseProcess.set event status.vi"("i ref in"=w625, "EventStatus"=w615, "error in (no error)"=w624) -> ("i ref out"=w610:refnum<vi>, "error out"=w612:errorcluster)  [unwired: 14 in, 1 out]
          n187 = Unbundle By Name(w612) -> ("source"=w620:string, "code"=w627:i32)
          n188 = call-poly "CoreLib.data 2 byte array.vi"("string"=w620) -> ("byteArray out"=w626:T1)  [unwired: 18 in]
          n189 = Bundle By Name(cluster=w617, "Data"=w626, "Error #"=w627, "Data Descriptor"="C:N") -> (w611:T2)
        }
        frame "Temp#EU" {
          n190 = call "CAEObj.unfold trend data.vi"("i ref in"=w670, "raw trend data"=w672) -> ("quality"=w665:i32, "timeStamp"=w664:dbl, "no link"=w662:bool, "i ref out"=w678:refnum<vi>, "data"=w677:i8[], "typeDescriptor"=w675:string, "error out"=w663:errorcluster)  [unwired: 9 in, 2 out]
          n191 = case shown="No Error" w663 {
            tunnel: [w690 w727] -> w681
            tunnel: w678 -> [w697 w727]
            tunnel: w674 -> [w696 w726]
            tunnel: [w689 w725] -> w680
            tunnel: w671 -> [_ w724]
            tunnel: w669 -> [w695 _]
            tunnel: w677 -> [w691 _]
            tunnel: w675 -> [_ _]
            tunnel: w665 -> [w688 _]
            tunnel: w664 -> [w686 _]
            tunnel: w662 -> [w685 _]
            frame No Error {
              n192 = To Time Stamp(1:w686) -> (0:w687:timestamp)
              n193 = call "CAEN_HVBoard.get data to modify.vi"("i ref in"=w697, "ms timeout (10000)"=w695, "error in (no error)"=w696) -> ("i ref out"=w694:refnum<vi>, "i attribute"=w684:T4, "error out"=w693:errorcluster)  [unwired: 13 in, 1 out]
              n194 = case "no link?" shown="False" w685 {
                selector: w685 -> [w698 w716]
                tunnel: [w702 w723] -> w692
                tunnel: w691 -> [_ w722]
                tunnel: w684 -> [w701 w721]
                tunnel: w688 -> [w700 w718]
                tunnel: w687 -> [w699 w717]
                tunnel: w684 -> [_ w715]
                frame True {
                  n195 = Bundle By Name(cluster=w701, "Temp#EU.DIM Status.quality"=w700, "Temp#EU.DIM Status.Time Stamp"=w699, "Temp#EU.DIM Status.no link"=w698) -> (w702:T4)
                }
                frame False {
                  n196 = Unbundle By Name(w715) -> ("Temp.Temp"=w710:dbl, "Temp#HighEU.Temp#HighEU"=w709:dbl, "Temp#LowEU.Temp#LowEU"=w708:dbl, "Temp#Multiplier"=w707:dbl)
                  n197 = Type Cast(x=w722) -> (*(type *) &x=w720:string)  [unwired: 1 in]
                  n198 = Build Array(w710, w709, w708) -> (w713:dbl[])
                  n199 = call "CAEN_HVSystem.EUString2UnitMultilier.vi"("EU String"=w720) -> ("Multiplier"=w706:dbl, "Unit"=w719:string)  [unwired: 2 in, 1 out]
                  n200 = Divide(x=w713, y=w707) -> (x/y=w714:dbl[])
                  n201 = Multiply(x=w714, y=w706) -> (x*y=w712:dbl[])
                  n202 = Index Array(array=w712, index #1=0 ("index")) -> (element #1=w705:dbl, element #2=w704:dbl, element #3=w703:dbl)  [unwired: 2 in]
                  n203 = Bundle By Name(cluster=w721, "Temp.Temp"=w705, "Temp#HighEU.Temp#HighEU"=w704, "Temp#LowEU.Temp#LowEU"=w703, "Temp#EU.DIM Status.quality"=w718, "Temp#EU.DIM Status.Time Stamp"=w717, "Temp#EU.Temp#EU"=w719, "Temp#Multiplier"=w706, "Temp#EU.DIM Status.no link"=w716) -> (w723:T4)
                }
              }
              n204 = call "CAEN_HVBoard.set modified data.vi"("i ref in"=w694, "i attribute"=w692, "error in (no error)"=w693) -> ("i ref out"=w690:refnum<vi>, "error out"=w689:errorcluster)  [unwired: 15 in]
            }
            frame Error {
              n205 = call "CoreLib.set data type mismatch.vi"("error in (no error)"=w726, "error source"=w724) -> ("error out"=w725:errorcluster)  [unwired: 17 in]
            }
          }
          n206 = call "BaseProcess.set event status.vi"("i ref in"=w681, "EventStatus"=w671, "error in (no error)"=w680) -> ("i ref out"=w666:refnum<vi>, "error out"=w668:errorcluster)  [unwired: 14 in, 1 out]
          n207 = Unbundle By Name(w668) -> ("source"=w676:string, "code"=w683:i32)
          n208 = call-poly "CoreLib.data 2 byte array.vi"("string"=w676) -> ("byteArray out"=w682:T1)  [unwired: 18 in]
          n209 = Bundle By Name(cluster=w673, "Data"=w682, "Error #"=w683, "Data Descriptor"="C:N") -> (w667:T2)
        }
        frame "Temp#HighEU" {
          n210 = call "CAEObj.unfold trend data.vi"("i ref in"=w736, "raw trend data"=w738) -> ("quality"=w730:i32, "timeStamp"=w729:dbl, "no link"=w728:bool, "i ref out"=w744:refnum<vi>, "data"=w743:i8[], "typeDescriptor"=w741:string, "error out"=w731:errorcluster)  [unwired: 9 in, 2 out]
          n211 = case shown="No Error" w731 {
            tunnel: [w757 w783] -> w747
            tunnel: w744 -> [w764 w783]
            tunnel: w740 -> [w763 w782]
            tunnel: [w756 w781] -> w746
            tunnel: w737 -> [_ w780]
            tunnel: w735 -> [w762 _]
            tunnel: w743 -> [w758 _]
            tunnel: w741 -> [_ _]
            tunnel: w730 -> [w753 _]
            tunnel: w729 -> [w752 _]
            tunnel: w728 -> [w750 _]
            frame No Error {
              n212 = To Time Stamp(1:w752) -> (0:w751:timestamp)
              n213 = call "CAEN_HVBoard.get data to modify.vi"("i ref in"=w764, "ms timeout (10000)"=w762, "error in (no error)"=w763) -> ("i ref out"=w761:refnum<vi>, "i attribute"=w755:T4, "error out"=w760:errorcluster)  [unwired: 13 in, 1 out]
              n214 = Unbundle By Name(w755) -> ("Temp#Multiplier"=w754:dbl)
              n215 = case "no link?" shown="False" w750 {
                selector: w750 -> [w765 w770]
                tunnel: [w769 w779] -> w759
                tunnel: w758 -> [_ w778]
                tunnel: w755 -> [w768 w776]
                tunnel: w754 -> [_ w774]
                tunnel: w753 -> [w767 w772]
                tunnel: w751 -> [w766 w771]
                frame True {
                  n216 = Bundle By Name(cluster=w768, "Temp#HighEU.DIM Status.quality"=w767, "Temp#HighEU.DIM Status.Time Stamp"=w766, "Temp#HighEU.DIM Status.no link"=w765) -> (w769:T4)
                }
                frame False {
                  n217 = Type Cast(type=0.0, x=w778) -> (*(type *) &x=w775:dbl)
                  n218 = Multiply(x=w774, y=w775) -> (x*y=w773:dbl)
                  n219 = Bundle By Name(cluster=w776, "Temp#HighEU.DIM Status.quality"=w772, "Temp#HighEU.DIM Status.Time Stamp"=w771, "Temp#HighEU.Temp#HighEU"=w773, "Temp#HighEU.DIM Status.no link"=w770) -> (w779:T4)
                }
              }
              n220 = call "CAEN_HVBoard.set modified data.vi"("i ref in"=w761, "i attribute"=w759, "error in (no error)"=w760) -> ("i ref out"=w757:refnum<vi>, "error out"=w756:errorcluster)  [unwired: 15 in]
            }
            frame Error {
              n221 = call "CoreLib.set data type mismatch.vi"("error in (no error)"=w782, "error source"=w780) -> ("error out"=w781:errorcluster)  [unwired: 17 in]
            }
          }
          n222 = call "BaseProcess.set event status.vi"("i ref in"=w747, "EventStatus"=w737, "error in (no error)"=w746) -> ("i ref out"=w732:refnum<vi>, "error out"=w734:errorcluster)  [unwired: 14 in, 1 out]
          n223 = Unbundle By Name(w734) -> ("source"=w742:string, "code"=w749:i32)
          n224 = call-poly "CoreLib.data 2 byte array.vi"("string"=w742) -> ("byteArray out"=w748:T1)  [unwired: 18 in]
          n225 = Bundle By Name(cluster=w739, "Data"=w748, "Error #"=w749, "Data Descriptor"="C:N") -> (w733:T2)
        }
        frame "Temp#LowEU" {
          n226 = call "CAEObj.unfold trend data.vi"("i ref in"=w792, "raw trend data"=w794) -> ("quality"=w786:i32, "timeStamp"=w785:dbl, "no link"=w784:bool, "i ref out"=w800:refnum<vi>, "data"=w799:i8[], "typeDescriptor"=w797:string, "error out"=w787:errorcluster)  [unwired: 9 in, 2 out]
          n227 = case shown="No Error" w787 {
            tunnel: [w813 w839] -> w803
            tunnel: w800 -> [w820 w839]
            tunnel: w796 -> [w819 w838]
            tunnel: [w812 w837] -> w802
            tunnel: w793 -> [_ w836]
            tunnel: w791 -> [w818 _]
            tunnel: w799 -> [w814 _]
            tunnel: w797 -> [_ _]
            tunnel: w786 -> [w809 _]
            tunnel: w785 -> [w808 _]
            tunnel: w784 -> [w806 _]
            frame No Error {
              n228 = To Time Stamp(1:w808) -> (0:w807:timestamp)
              n229 = call "CAEN_HVBoard.get data to modify.vi"("i ref in"=w820, "ms timeout (10000)"=w818, "error in (no error)"=w819) -> ("i ref out"=w817:refnum<vi>, "i attribute"=w811:T4, "error out"=w816:errorcluster)  [unwired: 13 in, 1 out]
              n230 = Unbundle By Name(w811) -> ("Temp#Multiplier"=w810:dbl)
              n231 = case "no link?" shown="False" w806 {
                selector: w806 -> [w821 w826]
                tunnel: [w825 w835] -> w815
                tunnel: w814 -> [_ w834]
                tunnel: w811 -> [w824 w832]
                tunnel: w810 -> [_ w830]
                tunnel: w809 -> [w823 w828]
                tunnel: w807 -> [w822 w827]
                frame True {
                  n232 = Bundle By Name(cluster=w824, "Temp#LowEU.DIM Status.quality"=w823, "Temp#LowEU.DIM Status.Time Stamp"=w822, "Temp#LowEU.DIM Status.no link"=w821) -> (w825:T4)
                }
                frame False {
                  n233 = Type Cast(type=0.0, x=w834) -> (*(type *) &x=w831:dbl)
                  n234 = Multiply(x=w830, y=w831) -> (x*y=w829:dbl)
                  n235 = Bundle By Name(cluster=w832, "Temp#LowEU.DIM Status.quality"=w828, "Temp#LowEU.DIM Status.Time Stamp"=w827, "Temp#LowEU.Temp#LowEU"=w829, "Temp#LowEU.DIM Status.no link"=w826) -> (w835:T4)
                }
              }
              n236 = call "CAEN_HVBoard.set modified data.vi"("i ref in"=w817, "i attribute"=w815, "error in (no error)"=w816) -> ("i ref out"=w813:refnum<vi>, "error out"=w812:errorcluster)  [unwired: 15 in]
            }
            frame Error {
              n237 = call "CoreLib.set data type mismatch.vi"("error in (no error)"=w838, "error source"=w836) -> ("error out"=w837:errorcluster)  [unwired: 17 in]
            }
          }
          n238 = call "BaseProcess.set event status.vi"("i ref in"=w803, "EventStatus"=w793, "error in (no error)"=w802) -> ("i ref out"=w788:refnum<vi>, "error out"=w790:errorcluster)  [unwired: 14 in, 1 out]
          n239 = Unbundle By Name(w790) -> ("source"=w798:string, "code"=w805:i32)
          n240 = call-poly "CoreLib.data 2 byte array.vi"("string"=w798) -> ("byteArray out"=w804:T1)  [unwired: 18 in]
          n241 = Bundle By Name(cluster=w795, "Data"=w804, "Error #"=w805, "Data Descriptor"="C:N") -> (w789:T2)
        }
        frame Default {
          # "In the default case, always call the ProcCase method of the parent class"
          n242 = call "DeviceBase.ProcCases.vi"("i ref in"=w841, "selector"=w842, "call cluster"=w843, "error in (no error)"=w846) -> ("i ref out"=w847:refnum<vi>, "answer cluster"=w844:T2, "error out"=w845:errorcluster)  [unwired: 13 in]
        }
      }
      n243 = case "Default?" shown="False" w13 {
        tunnel: w12 -> [w21 _]
        tunnel: w10 -> [w20 _]
        frame False {
          n244 = call "DeviceBase.set device state.vi"("i ref in"=w20, "implicit"=TRUE, "device error"=w21) -> ()  [unwired: 14 in, 3 out]
        }
        frame True {
        }
      }
    }
    frame Error {
    }
  }
  "answer cluster" <- w8
  "i ref out" <- w4
  "error out" <- w3
